vi "Climber Control.vi"() -> ()   [LabVIEW 2012]
uses:
  Globals/Shooter Elevation Positons.vi
  Globals/Useful Values.vi
  <vilib>/Rock Robotics/WPI/Joystick/WPI_JoystickGetSetRefNum.vi
panel:
  out "Motor Output":dbl
  out "Climbed":bool
  out "Pot Voltage":dbl
  in  "Stop At Value?":bool=TRUE
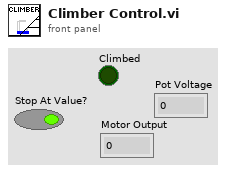
[diagram p1: front panel]
types:
  T1 = typedef "WPI_MotorControlDeviceRef.ctl" = cluster{"DeviceStatus":errorcluster, "Type":enum16{"PWM", "CAN"}, "PWM":cluster{"Digital Module":T2, "PWM Channel":T3, "DeadBand":T4}, "CAN":cluster{"Device Number":u8, "Control Mode":T5, "Semaphore":T6, "Max Vout":dbl}, "Invert":bool, "TransformRef":T7, "InvTransformRef":T7}
  T2 = typedef "FPGA_TypedefDigitalModule.ctl" = enum16{"Digital Module 1", "Digital Module 2"}
  T3 = typedef "FPGA_DIOPWMChannel.ctl" = enum8{"PWM 1", "PWM 2", "PWM 3", "PWM 4", "PWM 5", "PWM 6", "PWM 7", "PWM 8", "PWM 9", "PWM 10", "Invalid"}
  T4 = typedef "WPI_PWMDeadband.ctl" = cluster{"Name":string, "maxPositivePwm":i32, "minPositivePwm":i32, "centerPwm":i32, "maxNegativePwm":i32, "minNegativePwm":i32, "angularRange":u16}
  T5 = typedef "WPI_CANJaguar_ControlMode.ctl" = enum8{"Percent VBus", "Current", "Speed", "Position", "Voltage"}
  T6 = typedef "Semaphore RefNum" = refnum<k1>
  T7 = typedef "WPI_PWMTransform_ConPane.ctl" = refnum<vi>
  T8 = typedef "WPI_JoystickDevRef.ctl" = cluster{"Device":T9}
  T9 = typedef "WPI_JoystickDeviceEnum.ctl" = enum16{"USB 1", "USB 2", "USB 3", "USB 4", "Kinect 1", "Kinect 2"}
  T10 = typedef "WPI_AnalogChannelDevRef.ctl" = cluster{"DevStatus":errorcluster, "Analog Module":T11, "Analog Channel":T12}
  T11 = typedef "FPGA_TypedefAnalogModule.ctl" = enum16{"Analog Module 1", "Analog Module 2"}
  T12 = typedef "FPGA_AIChannel.ctl" = enum8{"AI 1", "AI 2", "AI 3", "AI 4", "AI 5", "AI 6", "AI 7", "AI 8", "Invalid"}
  T13 = typedef "WPI_JoystickButtonState.ctl" = cluster{"Button 1":bool, "Button 2":bool, "Button 3":bool, "Button 4":bool, "Button 5":bool, "Button 6":bool, "Button 7":bool, "Button 8":bool, "Button 9":bool, "Button 10":bool, "Button 11":bool, "Button 12":bool}
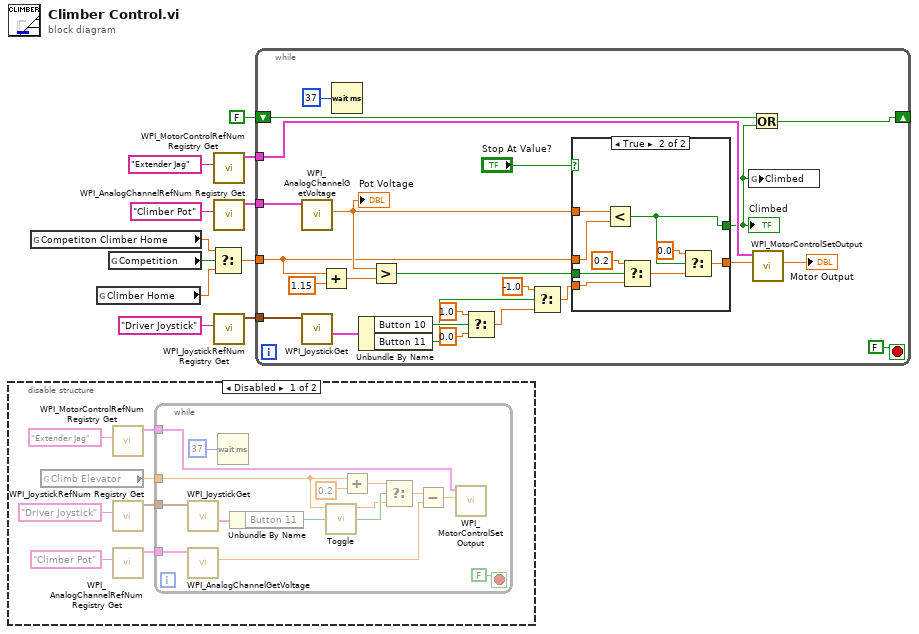
[diagram p0: block diagram]
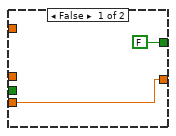
[diagram p3: hidden frame]
diagram:
  n1 = disable-structure shown="Disabled" {
    frame Disabled {
      n2 = global read "Shooter Elevation Positons.vi" "Climb Elevator"() -> (w12:dbl)
      n3 = call <vilib>:"WPI_MotorControlRefNum Registry Get.vi"("refnum name"="Extender Jag") -> ("MotorControlDevRef"=w15:T1)  [unwired: 9 in, 1 out]
      n4 = call <vilib>:"WPI_JoystickRefNum Registry Get.vi"("refnum name"="Driver Joystick") -> ("JoystickDevRef"=w16:T8)  [unwired: 9 in, 1 out]
      n5 = call <vilib>:"WPI_AnalogChannelRefNum Registry Get.vi"("refnum name"="Climber Pot") -> ("AIDeviceRef"=w13:T10)  [unwired: 9 in, 1 out]
      n6 = while {
        tunnel: w16 -> [w31]
        tunnel: w15 -> [w29]
        tunnel: w13 -> [w28]
        tunnel: w12 -> [w23]
        stop <- FALSE stop-if-true
        n7 = call <vilib>:"WPI_JoystickGet.vi"("JoystickDevRef"=w31) -> ("Buttons"=w30:T13)  [unwired: 4 in, 2 out]
        n8 = call <vilib>:"WPI_AnalogChannelGetVoltage.vi"("AIDeviceRef"=w28) -> ("Voltage"=w21:dbl)  [unwired: 8 in, 2 out]
        n9 = Wait (ms)(milliseconds to wait=u32 37) -> ()  [unwired: 1 out]
        n10 = Unbundle By Name(w30) -> ("Button 11"=w27:bool)
        n11 = call "Toggle.vi"("Input"=w27) -> ("Output"=w26:bool)
        n12 = Add(x=w23, y=0.2) -> (x+y=w24:dbl)
        n13 = Select(t=w24, s=w26, f=w23) -> (s? t:f=w22:dbl)
        n14 = Subtract(x=w22, y=w21) -> (x-y=w20:dbl)
        n15 = call <vilib>:"WPI_MotorControlSetOutput.vi"("Output"=w20, "MotorControlDevRef"=w29) -> ()  [unwired: 7 in, 3 out]
      }
    }
    frame Enabled {
    }
  }
  n16 = global read "Shooter Elevation Positons.vi" "Competiton Climber Home"() -> (w4:dbl)
  n17 = global read "Shooter Elevation Positons.vi" "Climber Home"() -> (w3:dbl)
  n18 = global read "Useful Values.vi" "Competition"() -> (w5:bool)
  n19 = Select(t=w4, s=w5, f=w3) -> (s? t:f=w2:dbl)
  n20 = call <vilib>:"WPI_MotorControlRefNum Registry Get.vi"("refnum name"="Extender Jag") -> ("MotorControlDevRef"=w8:T1)  [unwired: 9 in, 1 out]
  n21 = call <vilib>:"WPI_AnalogChannelRefNum Registry Get.vi"("refnum name"="Climber Pot") -> ("AIDeviceRef"=w6:T10)  [unwired: 9 in, 1 out]
  n22 = call <vilib>:"WPI_JoystickRefNum Registry Get.vi"("refnum name"="Driver Joystick") -> ("JoystickDevRef"=w9:T8)  [unwired: 9 in, 1 out]
  n23 = while {
    tunnel: w9 -> [w56]
    tunnel: w8 -> [w54]
    tunnel: w6 -> [w44]
    tunnel: w2 -> [w39]
    shift-right: [w34] -> _
    shift-left: FALSE -> [w33]
    stop <- FALSE stop-if-true
    n24 = call <vilib>:"WPI_AnalogChannelGetVoltage.vi"("AIDeviceRef"=w44) -> ("Voltage"=w40:dbl)  [unwired: 8 in, 2 out]
    "Pot Voltage" <- w40
    n25 = call <vilib>:"WPI_JoystickGet.vi"("JoystickDevRef"=w56) -> ("Buttons"=w55:T13)  [unwired: 4 in, 2 out]
    n26 = Add(x=w39, y=1.15) -> (x+y=w37:dbl)
    n27 = Wait (ms)(milliseconds to wait=u32 37) -> ()  [unwired: 1 out]
    n28 = Unbundle By Name(w55) -> ("Button 10"=w49:bool, "Button 11"=w47:bool)
    n29 = Greater?(x=w40, y=w37) -> (0:w42:bool)
    n30 = Select(t=1.0, s=w49, f=0.0) -> (s? t:f=w48:dbl)
    n31 = Select(t=-1.0, s=w47, f=w48) -> (s? t:f=w43:dbl)
    n32 = case shown="True" "Stop At Value?" {
      tunnel: w43 -> [w58 w67]
      tunnel: [w58 w61] -> w45
      tunnel: w42 -> [_ w65]
      tunnel: w40 -> [_ w64]
      tunnel: w39 -> [_ w60]
      tunnel: [FALSE w59] -> w35
      frame False {
      }
      frame True {
        n33 = Less?(x=w64, y=w60) -> (x < y?=w59:bool)
        n34 = Select(t=0.2, s=w65, f=w67) -> (s? t:f=w63:dbl)
        n35 = Select(t=0.0, s=w59, f=w63) -> (s? t:f=w61:dbl)
      }
    }
    "Climbed" <- w35
    n36 = global write "Useful Values.vi" "Climbed"(w35) -> ()
    n37 = Or(x=w33, y=w35) -> (x .or. y?=w34:bool)
    n38 = call <vilib>:"WPI_MotorControlSetOutput.vi"("Output"=w45, "MotorControlDevRef"=w54) -> ("Motor Output"=→"Motor Output":dbl)  [unwired: 7 in, 2 out]
  }
